vi "test-call.vi"() -> ()   [LabVIEW 2019]
uses:
  labview source/gRPC lv Support/grpc-lvsupport.lvlib
  <resource>/labview_grpc_server.dll
panel:
  out "Out":string
  out "Boolean":bool
  out "error out":errorcluster
  in  "Feature Toggle":string[](array[string])
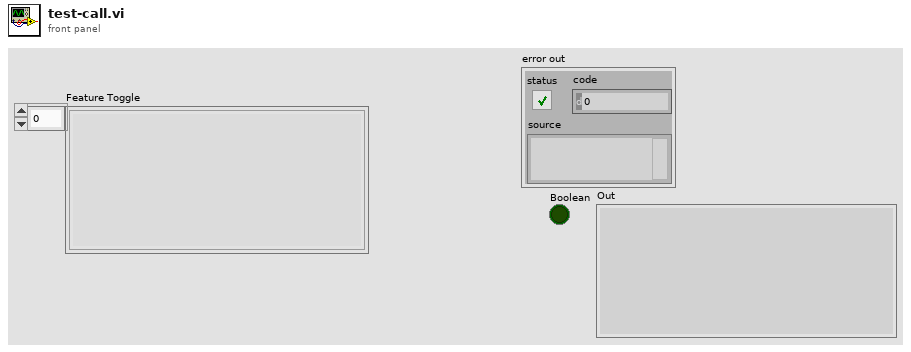
[diagram p1: front panel]
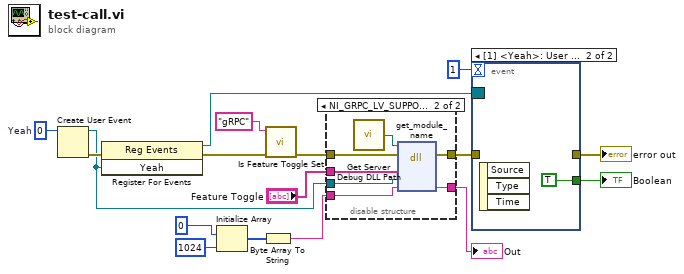
[diagram p0: block diagram]
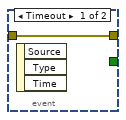
[diagram p2: hidden frame]
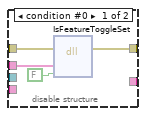
[diagram p3: hidden frame]
diagram:
  w14 = 0  # Yeah
  n1 = Create User Event(user event datatype=w14) -> (user event=w7:refnum<user-event>, error out=w13:errorcluster)  [unwired: 1 in]
  n2 = register-events(error in=w13, w7) -> (reference out=w8:refnum<event-registration>, error out=w12:errorcluster)  [unwired: 1 in]
  n3 = Initialize Array(u8 0, 1024 ("dimension size")) -> (w5:u8[])
  n4 = Byte Array To String(unsigned byte array=w5) -> (string=w4:string)
  n5 = call "Is Feature Toggle Set.vi"("error in (no error)"=w12, "Feature Toggle"="gRPC" ("Module Path")) -> ("error out"=w15:errorcluster)  [unwired: 8 in, 1 out]
  n6 = disable-structure shown="NI_GRPC_LV_SUPPORT_DEBUG==True&&RUN_TIME_ENGINE==False" {
    disable-tunnel: [w21 w29] -> w11
    disable-tunnel: w15 -> [w19 w28]
    disable-tunnel: "Feature Toggle" -> [w18 w27]
    disable-tunnel: w7 -> [_ w25]
    disable-tunnel: w4 -> [_ w24]
    disable-tunnel: [_ w23] -> w1
    frame condition #0 {
      n7 = dll-call lib="C:/Program Files (x86)/National Instruments/LabVIEW 2024/resource/labview_grpc_server.*" fn="IsFeatureToggleSet"(error in=w19, "Feature"=w18, "isSet"=FALSE) -> (error out=w21:errorcluster, "isSet"=w22:bool)  [unwired: 4 in, 1 out]
    }
    frame condition #1 (active) {
      n8 = call "Get Server Debug DLL Path.vi"() -> ("Server Debug DLL Path"=w26:path)
      n9 = dll-call lib="?" fn="get_module_name"(path in=w26, error in=w28, "Names"=w27, "Ref"=w25, "Out"=w24) -> (error out=w29:errorcluster, "Out"=w23:string)  [unwired: 4 in, 1 out]
    }
  }
  "Out" <- w1
  n10 = event shown="[1] <Yeah>: User Event" {
    selector: w8 -> [_ _]
    dyn-events: _ -> [_ _]
    timeout: 1 -> [_ _]
    tunnel: [w30 _] -> w9
    tunnel: w11 -> [w30 _]
    tunnel: [_ TRUE] -> w2
    event Timeout {
      n11 = event-data() -> ()  [unwired: 1 in, 3 out]
    }
    event User Event {
      n12 = event-data() -> ()  [unwired: 1 in, 3 out]
    }
  }
  "error out" <- w9
  "Boolean" <- w2
